vi "Stop Device.vi"(8 "error in (no error)":errorcluster, 10 "device":string, 11 "Device Manager in":refnum<class "Device Manager.lvclass">) -> (0 "error out":errorcluster, 2 "device not found?":bool, 3 "Device Manager out":refnum<class "Device Manager.lvclass">)   [LabVIEW 2020, in "Device Manager.lvclass"]
uses:
  Device Manager.lvclass
  Device/Device Messages/Stop Action Msg/Stop Action Msg.lvclass
  Device/Device Messages/Clear Action Msg/Clear Action Msg.lvclass
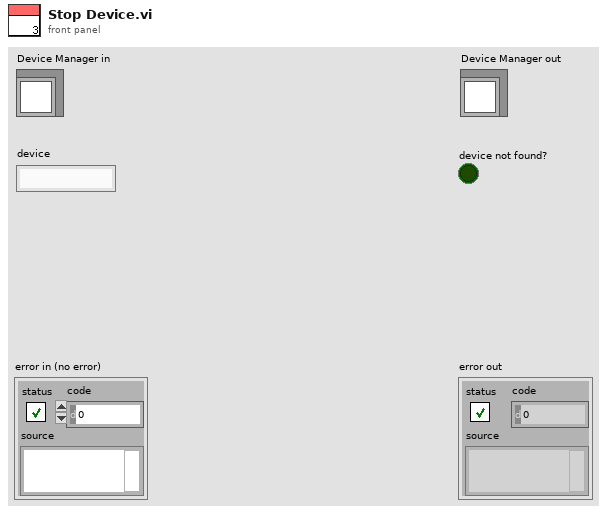
[diagram p1: front panel]
types:
  T1 = map{string, refnum<class "Message Enqueuer.lvclass">}
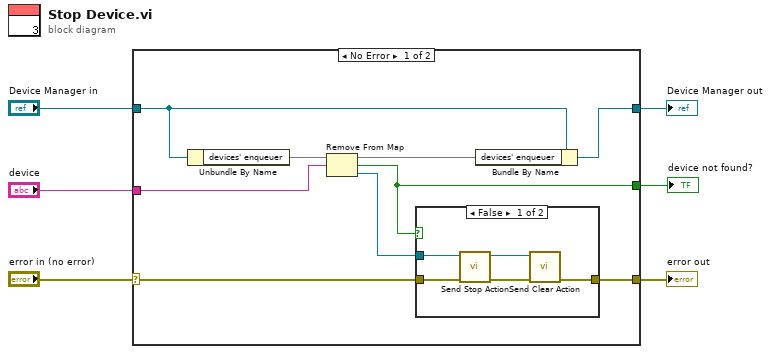
[diagram p0: block diagram]
diagram:
  n1 = case shown="No Error" "error in (no error)" {
    selector: "error in (no error)" -> [w10 w23]
    tunnel: [w7 w23] -> w5
    tunnel: [w11 w22] -> w3
    tunnel: "Device Manager in" -> [w13 w22]
    tunnel: "device" -> [w14 _]
    tunnel: [w8 _] -> w1
    frame No Error {
      n2 = Unbundle By Name(w13) -> ("devices' enqueuer"=w15:T1)
      n3 = Remove From Map(10:w14, 11:w15) -> (1:w9:refnum<class "Message Enqueuer.lvclass">, 2:w8:bool, 3:w12:T1)
      n4 = case shown="False" w8 {
        tunnel: w10 -> [w20 w21]
        tunnel: w9 -> [w19 _]
        tunnel: [w16 w21] -> w7
        frame False {
          n5 = call "Send Stop Action.vi"("error in (no error)"=w20, "Message Enqueuer"=w19) -> ("error out"=w18:errorcluster, "Message Enqueuer out"=w17:refnum<class "Message Enqueuer.lvclass">)  [unwired: 8 in]
          n6 = call "Send Clear Action.vi"("error in (no error)"=w18, "Message Enqueuer"=w17) -> ("error out"=w16:errorcluster)  [unwired: 8 in, 1 out]
        }
        frame True {
        }
      }
      n7 = Bundle By Name(cluster=w13, "devices' enqueuer"=w12) -> (w11:refnum<class "Device Manager.lvclass">)
    }
    frame Error {
    }
  }
  "error out" <- w5
  "Device Manager out" <- w3
  "device not found?" <- w1
